vi "Individual Tube ON - OFF.vi"(6 "Single Tube ON/OFF":bool, 7 "Tube #":i32 min=0 max=63, 11 "First Tube Number":i32 min=0 max=63) -> ()   [LabVIEW 2020]
uses:
  <vilib>/DAQmx/write.llb/DAQmx Write (Digital U8 1Chan 1Samp).vi
  <vilib>/DAQmx/create/channels.llb/DAQmx Create Channel (DO-Digital Output).vi
  <vilib>/DAQmx/miscellaneous.llb/DAQmx Fill In Error Info.vi
panel:
  out "Status(U8)":u8
  in  "lines":tag="Dev2/port0/line0:7"
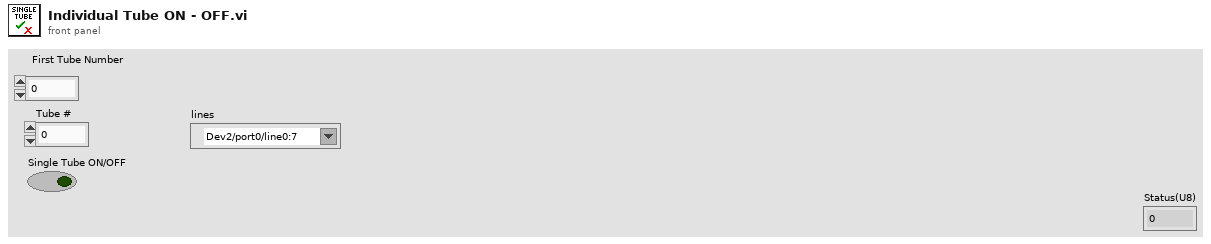
[diagram p1: front panel]
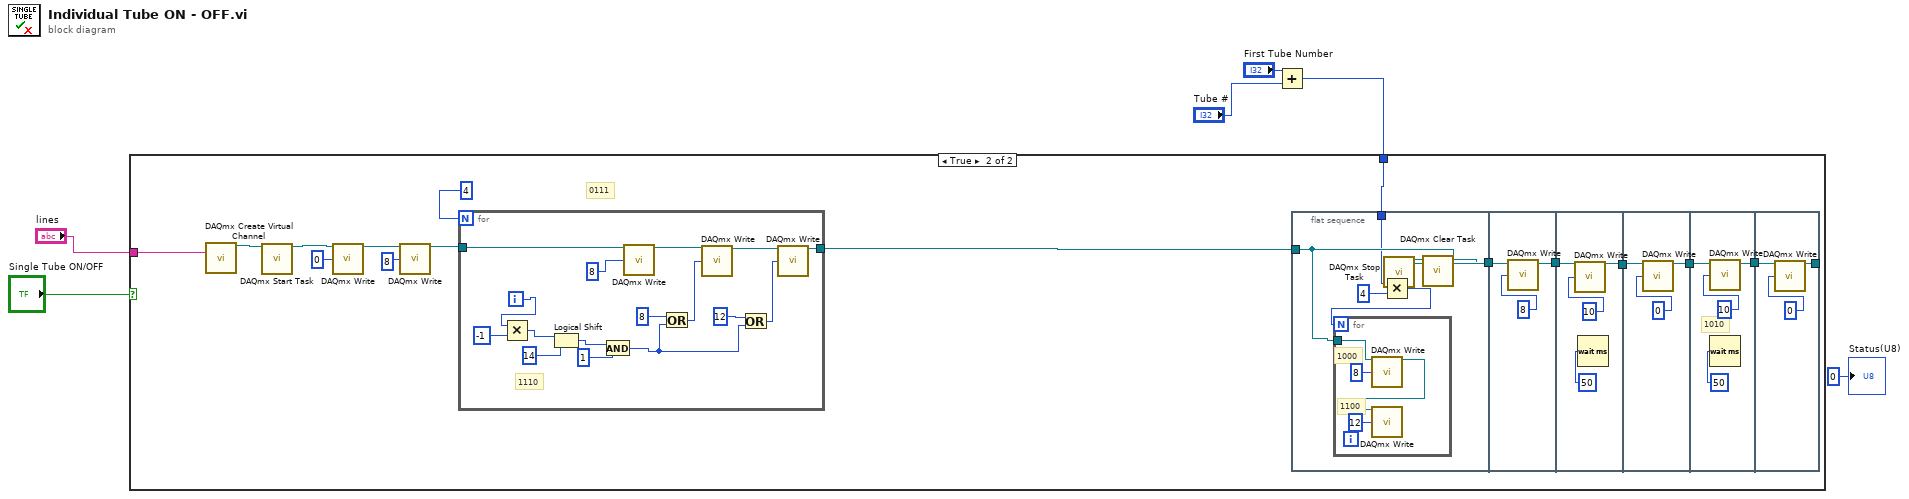
[diagram p0: block diagram]
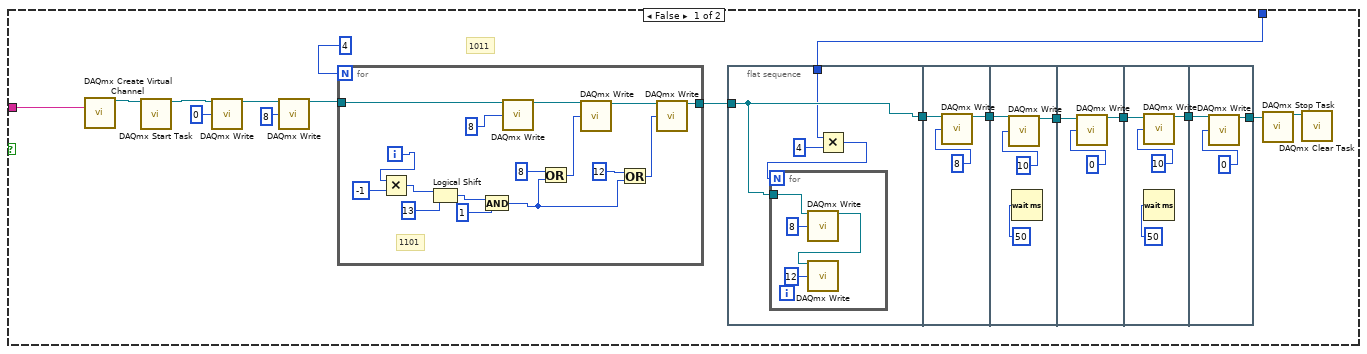
[diagram p2: hidden frame]
diagram:
  n1 = Add(x="First Tube Number", y="Tube #") -> (x+y=w1:i32)
  n2 = case shown="True" "Single Tube ON/OFF" {
    tunnel: w1 -> [w8 w66]
    tunnel: "lines" -> [w7 w65]
    frame False {
      # "1011"
      n3 = call-poly <vilib>:"DAQmx Create Virtual Channel.vi"("lines"=w7) -> ("task out"=w18:refnum<k21>)  [unwired: 13 in, 1 out]
      n4 = call <vilib>:"DAQmx Start Task.vi"("task/channels in"=w18) -> ("task out"=w13:refnum<k21>)  [unwired: 13 in, 1 out]
      n5 = call-poly <vilib>:"DAQmx Write.vi"("task/channels in"=w13, "data"=u8 0) -> ("task out"=w12:refnum<k21>)  [unwired: 11 in, 2 out]
      n6 = call-poly <vilib>:"DAQmx Write.vi"("task/channels in"=w12, "data"=u8 8) -> ("task out"=w15:refnum<k21>)  [unwired: 11 in, 2 out]
      n7 = for {
        N: 4 -> [_]
        tunnel: w15 -> [w53]
        tunnel: [w50] -> w9
        i -> [w62]
        # "1101"
        n8 = Multiply(x=w62, y=-1) -> (x*y=w60:i32)
        n9 = Logical Shift(y=w60, x=u8 13) -> (x << y=w64:u8)
        n10 = And(x=w64, y=u32 1) -> (x .and. y?=w56:u32)
        n11 = call-poly <vilib>:"DAQmx Write.vi"("task/channels in"=w53, "data"=u32 8 ("x")) -> ("task out"=w52:refnum<k21>)  [unwired: 11 in, 2 out]
        n12 = Or(x=u32 8, y=w56) -> (x .or. y?=w57:u32)
        n13 = call-poly <vilib>:"DAQmx Write.vi"("task/channels in"=w52, "data"=w57) -> ("task out"=w51:refnum<k21>)  [unwired: 11 in, 2 out]
        n14 = Or(x=u32 12, y=w56) -> (x .or. y?=w54:u32)
        n15 = call-poly <vilib>:"DAQmx Write.vi"("task/channels in"=w51, "data"=w54) -> ("task out"=w50:refnum<k21>)  [unwired: 11 in, 2 out]
      }
      n16 = flat-sequence {
        tunnel: [w25] -> w23
        tunnel: w9 -> [w25]
        tunnel: w8 -> [w24]
        tunnel: [w32] -> w22
        tunnel: w23 -> [w33]
        tunnel: w22 -> [w36]
        tunnel: [w35] -> w21
        tunnel: w21 -> [w40]
        tunnel: [w39] -> w20
        tunnel: w20 -> [w43]
        tunnel: [w42] -> w19
        tunnel: w19 -> [w47]
        tunnel: [w46] -> w10
        frame #0 {
          n17 = Multiply(x=w24, y=4) -> (x*y=w27:i32)
          n18 = for {
            N: w27 -> [_]
            tunnel: w25 -> [w29]
            n19 = call-poly <vilib>:"DAQmx Write.vi"("task/channels in"=w29, "data"=u8 8) -> ("task out"=w28:refnum<k21>)  [unwired: 11 in, 2 out]
            n20 = call-poly <vilib>:"DAQmx Write.vi"("task/channels in"=w28, "data"=u8 12) -> ()  [unwired: 11 in, 3 out]
          }
        }
        frame #1 {
          n21 = call-poly <vilib>:"DAQmx Write.vi"("task/channels in"=w33, "data"=u8 8) -> ("task out"=w32:refnum<k21>)  [unwired: 11 in, 2 out]
        }
        frame #2 {
          n22 = call-poly <vilib>:"DAQmx Write.vi"("task/channels in"=w36, "data"=u8 10) -> ("task out"=w35:refnum<k21>)  [unwired: 11 in, 2 out]
          n23 = Wait (ms)(milliseconds to wait=u32 50) -> ()  [unwired: 1 out]
        }
        frame #3 {
          n24 = call-poly <vilib>:"DAQmx Write.vi"("task/channels in"=w40, "data"=u8 0) -> ("task out"=w39:refnum<k21>)  [unwired: 11 in, 2 out]
        }
        frame #4 {
          n25 = call-poly <vilib>:"DAQmx Write.vi"("task/channels in"=w43, "data"=u8 10) -> ("task out"=w42:refnum<k21>)  [unwired: 11 in, 2 out]
          n26 = Wait (ms)(milliseconds to wait=u32 50) -> ()  [unwired: 1 out]
        }
        frame #5 {
          n27 = call-poly <vilib>:"DAQmx Write.vi"("task/channels in"=w47, "data"=u8 0) -> ("task out"=w46:refnum<k21>)  [unwired: 11 in, 2 out]
        }
      }
      n28 = call <vilib>:"DAQmx Stop Task.vi"("task/channels in"=w10) -> ("task out"=w17:refnum<k21>)  [unwired: 13 in, 1 out]
      n29 = call <vilib>:"DAQmx Clear Task.vi"("task in"=w17) -> ()  [unwired: 14 in, 1 out]
    }
    frame True {
      # "0111"
      n30 = call-poly <vilib>:"DAQmx Create Virtual Channel.vi"("lines"=w65) -> ("task out"=w76:refnum<k21>)  [unwired: 13 in, 1 out]
      n31 = call <vilib>:"DAQmx Start Task.vi"("task/channels in"=w76) -> ("task out"=w71:refnum<k21>)  [unwired: 13 in, 1 out]
      n32 = call-poly <vilib>:"DAQmx Write.vi"("task/channels in"=w71, "data"=u8 0) -> ("task out"=w70:refnum<k21>)  [unwired: 11 in, 2 out]
      n33 = call-poly <vilib>:"DAQmx Write.vi"("task/channels in"=w70, "data"=u8 8) -> ("task out"=w73:refnum<k21>)  [unwired: 11 in, 2 out]
      n34 = for {
        N: 4 -> [_]
        tunnel: w73 -> [w111]
        tunnel: [w108] -> w67
        i -> [w120]
        # "1110"
        n35 = Multiply(x=w120, y=-1) -> (x*y=w118:i32)
        n36 = Logical Shift(y=w118, x=u8 14) -> (x << y=w122:u8)
        n37 = And(x=w122, y=u32 1) -> (x .and. y?=w114:u32)
        n38 = call-poly <vilib>:"DAQmx Write.vi"("task/channels in"=w111, "data"=u32 8 ("x")) -> ("task out"=w110:refnum<k21>)  [unwired: 11 in, 2 out]
        n39 = Or(x=u32 8, y=w114) -> (x .or. y?=w115:u32)
        n40 = call-poly <vilib>:"DAQmx Write.vi"("task/channels in"=w110, "data"=w115) -> ("task out"=w109:refnum<k21>)  [unwired: 11 in, 2 out]
        n41 = Or(x=u32 12, y=w114) -> (x .or. y?=w112:u32)
        n42 = call-poly <vilib>:"DAQmx Write.vi"("task/channels in"=w109, "data"=w112) -> ("task out"=w108:refnum<k21>)  [unwired: 11 in, 2 out]
      }
      n43 = flat-sequence {
        tunnel: [w83] -> w81
        tunnel: w67 -> [w83]
        tunnel: w66 -> [w82]
        tunnel: [w90] -> w80
        tunnel: w81 -> [w91]
        tunnel: w80 -> [w94]
        tunnel: [w93] -> w79
        tunnel: w79 -> [w98]
        tunnel: [w97] -> w78
        tunnel: w78 -> [w101]
        tunnel: [w100] -> w77
        tunnel: w77 -> [w105]
        tunnel: [w104] -> w68
        frame #0 {
          n44 = Multiply(x=w82, y=4) -> (x*y=w85:i32)
          n45 = for {
            N: w85 -> [_]
            tunnel: w83 -> [w87]
            # "1100"
            # "1000"
            n46 = call-poly <vilib>:"DAQmx Write.vi"("task/channels in"=w87, "data"=u8 8) -> ("task out"=w86:refnum<k21>)  [unwired: 11 in, 2 out]
            n47 = call-poly <vilib>:"DAQmx Write.vi"("task/channels in"=w86, "data"=u8 12) -> ()  [unwired: 11 in, 3 out]
          }
        }
        frame #1 {
          n48 = call-poly <vilib>:"DAQmx Write.vi"("task/channels in"=w91, "data"=u8 8) -> ("task out"=w90:refnum<k21>)  [unwired: 11 in, 2 out]
        }
        frame #2 {
          n49 = call-poly <vilib>:"DAQmx Write.vi"("task/channels in"=w94, "data"=u8 10) -> ("task out"=w93:refnum<k21>)  [unwired: 11 in, 2 out]
          n50 = Wait (ms)(milliseconds to wait=u32 50) -> ()  [unwired: 1 out]
        }
        frame #3 {
          n51 = call-poly <vilib>:"DAQmx Write.vi"("task/channels in"=w98, "data"=u8 0) -> ("task out"=w97:refnum<k21>)  [unwired: 11 in, 2 out]
        }
        frame #4 {
          # "1010"
          n52 = call-poly <vilib>:"DAQmx Write.vi"("task/channels in"=w101, "data"=u8 10) -> ("task out"=w100:refnum<k21>)  [unwired: 11 in, 2 out]
          n53 = Wait (ms)(milliseconds to wait=u32 50) -> ()  [unwired: 1 out]
        }
        frame #5 {
          n54 = call-poly <vilib>:"DAQmx Write.vi"("task/channels in"=w105, "data"=u8 0) -> ("task out"=w104:refnum<k21>)  [unwired: 11 in, 2 out]
        }
      }
      n55 = call <vilib>:"DAQmx Stop Task.vi"("task/channels in"=w68) -> ("task out"=w75:refnum<k21>)  [unwired: 13 in, 1 out]
      n56 = call <vilib>:"DAQmx Clear Task.vi"("task in"=w75) -> ()  [unwired: 14 in, 1 out]
    }
  }
  "Status(U8)" <- u8 0
